vi "Autonomous Independent.vi"() -> ()   [LabVIEW 2015]
doc: "This VI is called when autonomous begins, and will automatically be terminated when autonomous ends. You can carry out timed or sensor driven robot movement independently without needing to return to the caller."
uses:
  <vilib>/Rock Robotics/WPI/Utilities/WPI_GetSetVariantRefNum.vi
  <vilib>/Rock Robotics/Network Tables/NT Read String.vi
  <vilib>/Rock Robotics/WPI/RobotDrive/WPI_RobotDriveArcadeDrive_Standard(NoSaturation).vi
  <vilib>/Rock Robotics/Network Tables/NT Write Numeric Array.vi
panel:
  out "Current Movement, for debugging":T1 {"Y Joystick Value" scale=1.0..-1.0; "X Joystick Value" scale=-1.0..1.0}
  in  "Array of robot movements":T2(array[cluster])=[{"X Joystick Value"=0.39393939393939403, "Y Joystick Value"=0.0, "Delay (sec)"=1.0, "Movement Name"="turn"}, {"X Joystick Value"=-0.3737373737373737, "Y Joystick Value"=0.0, "Delay (sec)"=1.0, "Movement Name"="turn back"}] {"Y Joystick Value" scale=1.0..-1.0; "X Joystick Value" scale=-1.0..1.0}
  # "Be sure to right-click and choose Data Operations>>Make Current Value default if you want to save the array values with the VI"
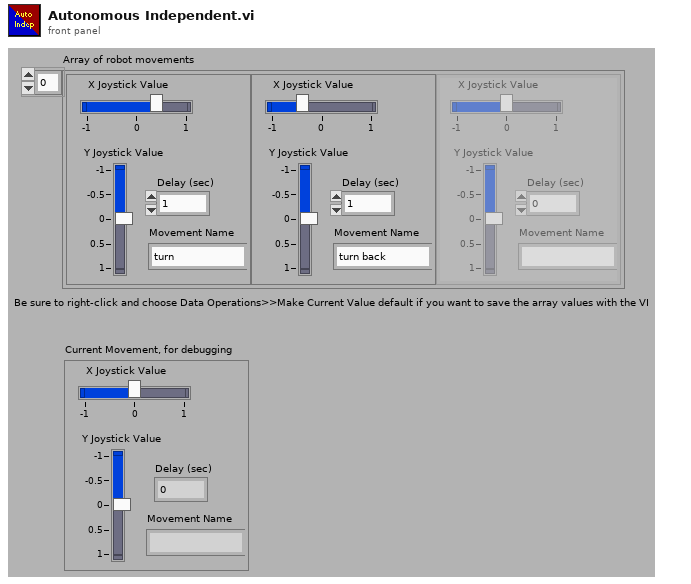
[diagram p1: front panel]
types:
  T1 = cluster{"X Joystick Value":dbl, "Y Joystick Value":dbl, "Delay (sec)":dbl, "Movement Name":string}
  T2 = cluster{"X Joystick Value":dbl, "Y Joystick Value":dbl, "Delay (sec)":dbl, "Movement Name":string}[]
  T3 = typedef "WPI_JoystickDevRef.ctl" = cluster{"Device":T4}
  T4 = typedef "WPI_JoystickDeviceEnum.ctl" = enum16{"USB 0", "USB 1", "USB 2", "USB 3", "USB 4", "USB 5"}
  T5 = typedef "WPI_RobotDriveDevRef.ctl" = cluster{"DevStatus":errorcluster, "Motors[]":T6[], "Square Inputs":bool, "Max Output":dbl}
  T6 = typedef "WPI_MotorControlDeviceRef.ctl" = cluster{"DeviceStatus":errorcluster, "Type":T7, "PWM":cluster{"PWM Channel":T8, "DeadBand":T9}, "CAN":cluster{"Device Number":u8, "Control Mode":T10, "Semaphore":T11, "Max Vout":dbl, "TalonSRX Control Mode":T12}, "Invert":bool}
  T7 = typedef "WPI_MotorControlType.ctl" = enum16{"PWM", "CAN", "CANTalonSRX"}
  T8 = typedef "FPGA_DIOPWMChannel.ctl" = enum8{"PWM 0", "PWM 1", "PWM 2", "PWM 3", "PWM 4", "PWM 5", "PWM 6", "PWM 7", "PWM 8", "PWM 9", "PWM MXP 0", "PWM MXP 1", "PWM MXP 2", "PWM MXP 3", "PWM MXP 4", "PWM MXP 5", "PWM MXP 6", "PWM MXP 7", "PWM MXP 8", "PWM MXP 9", "Invalid"}
  T9 = typedef "WPI_PWMDeadband.ctl" = cluster{"Name":string, "maxPositivePwm":i32, "minPositivePwm":i32, "centerPwm":i32, "maxNegativePwm":i32, "minNegativePwm":i32, "angularRange":u16}
  T10 = typedef "WPI_CANJaguar_ControlMode.ctl" = enum8{"Percent VBus", "Current", "Speed", "Position", "Voltage"}
  T11 = typedef "Semaphore RefNum" = refnum<k1>
  T12 = typedef "WPI_CANTalonSRX_APIControlMode.ctl" = enum8{"Percent VBus", "Speed", "Position", "Slave", "Unchanged / Invalid", "Voltage Compensation", "Current", "Motion Profile"}
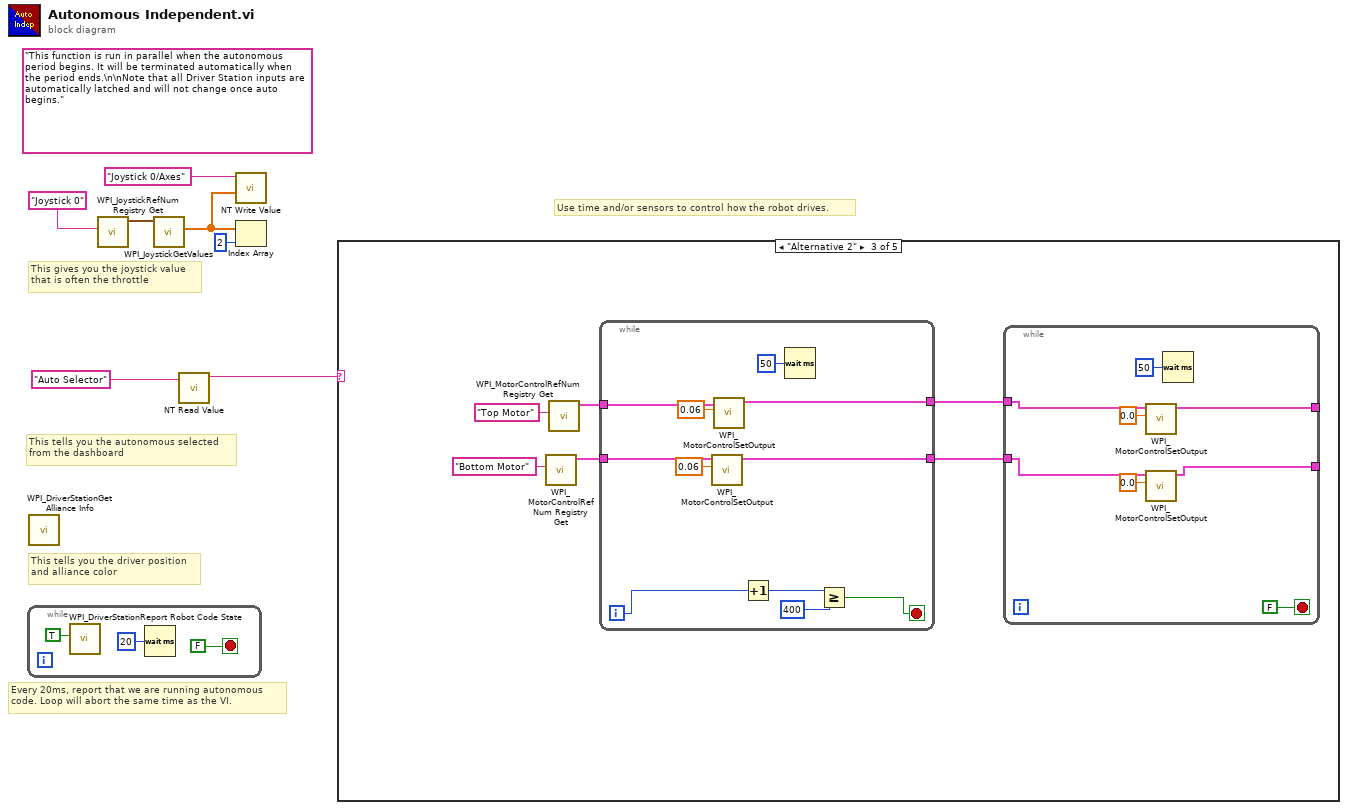
[diagram p0: block diagram]
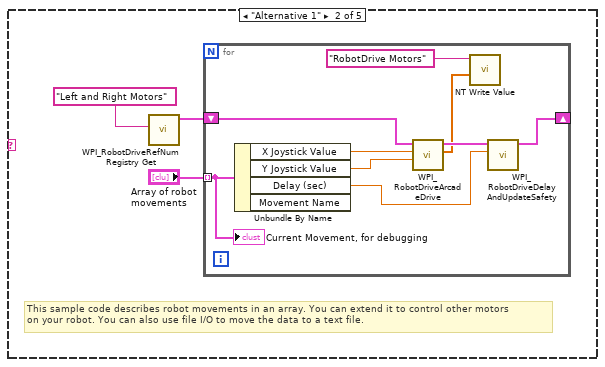
[diagram p3: hidden frame]
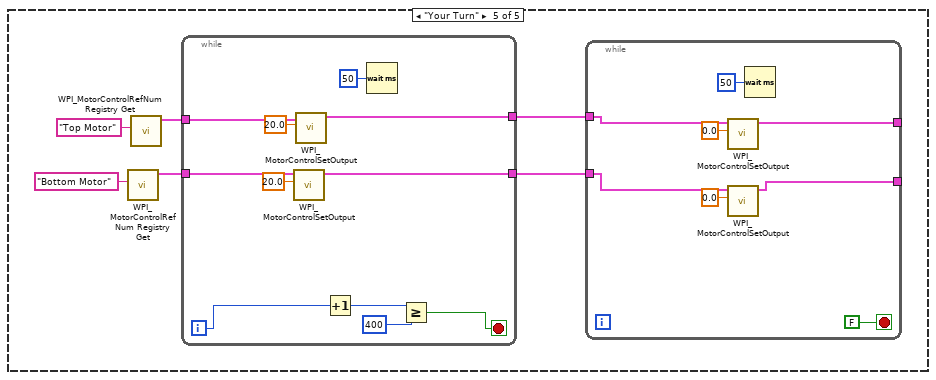
[diagram p5: hidden frame]
diagram:
  (unwired) "This function is run in parallel when the autonomous period begins. It will be terminated automatically when the period ends.\n\nNote that all Driver Station inputs are automatically latched and will not change once auto begins."
  # "This tells you the autonomous selected\nfrom the dashboard"
  # "Every 20ms, report that we are running autonomous\ncode. Loop will abort the same time as the VI."
  # "This gives you the joystick value\nthat is often the throttle"
  # "Use time and/or sensors to control how the robot drives."
  # "This tells you the driver position\nand alliance color"
  n1 = while {
    stop <- FALSE stop-if-true
    n2 = call <vilib>:"WPI_DriverStationReport Robot Code State.vi"("Autonomous"=TRUE) -> ()  [unwired: 10 in, 1 out]
    n3 = Wait (ms)(milliseconds to wait=u32 20) -> ()  [unwired: 1 out]
  }
  n4 = call <vilib>:"WPI_DriverStationGet Alliance Info.vi"() -> ()  [unwired: 12 out]
  n5 = call <vilib>:"WPI_JoystickRefNum Registry Get.vi"("refnum name"="Joystick 0") -> ("JoystickDevRef"=w6:T3)  [unwired: 1 in, 9 out]
  n6 = call <vilib>:"WPI_JoystickGetValues.vi"("JoystickDevRef"=w6) -> ("Axes"=w2:dbl[])  [unwired: 6 in, 4 out]
  n7 = call-poly <vilib>:"NT Read Value.vi"("Name"="Auto Selector") -> ("String"=w3:string)  [unwired: 9 in, 1 out]
  n8 = call-poly <vilib>:"NT Write Value.vi"("Numeric Array"=w2, "Name"="Joystick 0/Axes") -> ()  [unwired: 9 in, 1 out]
  n9 = Index Array(array=w2, index=2) -> ()  [unwired: 1 out]
  n10 = case shown="\"Alternative 2\"" w3 {
    frame Default {
      # "You can put your main auto here, or you can right-click on the case and make any\nother frame be the default case."
      # "This is the frame that will execute if no selection is made, or if it is not recognized"
    }
    frame "Alternative 1" {
      # "This sample code describes robot movements in an array. You can extend it to control other motors\non your robot. You can also use file I/O to move the data to a text file."
      n11 = call <vilib>:"WPI_RobotDriveRefNum Registry Get.vi"("refnum name"="Left and Right Motors") -> ("RobotDriveDevRef"=w12:T5)  [unwired: 1 in, 9 out]
      n12 = for {
        shift-right: [w20] -> _
        shift-left: w12 -> [w21]
        tunnel: "Array of robot movements" -> [w16] mode=indexing
        n13 = Unbundle By Name(w16) -> ("X Joystick Value"=w19:dbl, "Y Joystick Value"=w18:dbl, "Delay (sec)"=w17:dbl)  [unwired: 1 out]
        n14 = call-poly <vilib>:"WPI_RobotDriveArcadeDrive.vi"("Y axis value"=w18, "X axis value"=w19, "RobotDriveDevRef"=w21) -> ("Motor Values"=w14:dbl[], "RobotDriveDevRef"=w22:T5)  [unwired: 1 in, 6 out]
        n15 = call-poly <vilib>:"NT Write Value.vi"("Numeric Array"=w14, "Name"="RobotDrive Motors") -> ()  [unwired: 9 in, 1 out]
        n16 = call <vilib>:"WPI_RobotDriveDelayAndUpdateSafety.vi"("Delay (s)"=w17, "RobotDriveDevRef"=w22) -> ("RobotDriveDevRef 2"=w20:T5)  [unwired: 8 in, 1 out]
        "Current Movement, for debugging" <- w16
      }
    }
    frame "Alternative 2" {
      n17 = call <vilib>:"WPI_MotorControlRefNum Registry Get.vi"("refnum name"="Bottom Motor") -> ("MotorControlDevRef"=w28:T6)  [unwired: 9 in, 1 out]
      n18 = call <vilib>:"WPI_MotorControlRefNum Registry Get.vi"("refnum name"="Top Motor") -> ("MotorControlDevRef"=w27:T6)  [unwired: 9 in, 1 out]
      n19 = while {
        tunnel: w28 -> [w47]
        tunnel: w27 -> [w46]
        tunnel: [w40] -> w24
        tunnel: [w39] -> w23
        i -> [w42]
        stop <- w43 stop-if-true
        n20 = call <vilib>:"WPI_MotorControlSetOutput.vi"("Output"=0.06, "MotorControlDevRef"=w47) -> ("MotorControlDevRef"=w39:T6)  [unwired: 7 in, 2 out]
        n21 = call <vilib>:"WPI_MotorControlSetOutput.vi"("Output"=0.06, "MotorControlDevRef"=w46) -> ("MotorControlDevRef"=w40:T6)  [unwired: 7 in, 2 out]
        n22 = Increment(x=w42) -> (x+1=w44:i32)
        n23 = Wait (ms)(milliseconds to wait=u32 50) -> ()  [unwired: 1 out]
        n24 = Greater Or Equal?(x=w44, y=400) -> (x >= y?=w43:bool)
      }
      n25 = while {
        tunnel: w24 -> [w34]
        tunnel: w23 -> [w32]
        tunnel: [w33] -> _
        tunnel: [w31] -> _
        stop <- FALSE stop-if-true
        n26 = call <vilib>:"WPI_MotorControlSetOutput.vi"("Output"=0.0, "MotorControlDevRef"=w34) -> ("MotorControlDevRef"=w33:T6)  [unwired: 7 in, 2 out]
        n27 = call <vilib>:"WPI_MotorControlSetOutput.vi"("Output"=0.0, "MotorControlDevRef"=w32) -> ("MotorControlDevRef"=w31:T6)  [unwired: 7 in, 2 out]
        n28 = Wait (ms)(milliseconds to wait=u32 50) -> ()  [unwired: 1 out]
      }
    }
    frame "Alternative 3" {
    }
    frame "Your Turn" {
      n29 = call <vilib>:"WPI_MotorControlRefNum Registry Get.vi"("refnum name"="Bottom Motor") -> ("MotorControlDevRef"=w53:T6)  [unwired: 9 in, 1 out]
      n30 = call <vilib>:"WPI_MotorControlRefNum Registry Get.vi"("refnum name"="Top Motor") -> ("MotorControlDevRef"=w52:T6)  [unwired: 9 in, 1 out]
      n31 = while {
        tunnel: w53 -> [w72]
        tunnel: w52 -> [w71]
        tunnel: [w65] -> w49
        tunnel: [w64] -> w48
        i -> [w67]
        stop <- w68 stop-if-true
        n32 = call <vilib>:"WPI_MotorControlSetOutput.vi"("Output"=20.0, "MotorControlDevRef"=w72) -> ("MotorControlDevRef"=w64:T6)  [unwired: 7 in, 2 out]
        n33 = call <vilib>:"WPI_MotorControlSetOutput.vi"("Output"=20.0, "MotorControlDevRef"=w71) -> ("MotorControlDevRef"=w65:T6)  [unwired: 7 in, 2 out]
        n34 = Increment(x=w67) -> (x+1=w69:i32)
        n35 = Wait (ms)(milliseconds to wait=u32 50) -> ()  [unwired: 1 out]
        n36 = Greater Or Equal?(x=w69, y=400) -> (x >= y?=w68:bool)
      }
      n37 = while {
        tunnel: w49 -> [w59]
        tunnel: w48 -> [w57]
        tunnel: [w58] -> _
        tunnel: [w56] -> _
        stop <- FALSE stop-if-true
        n38 = call <vilib>:"WPI_MotorControlSetOutput.vi"("Output"=0.0, "MotorControlDevRef"=w59) -> ("MotorControlDevRef"=w58:T6)  [unwired: 7 in, 2 out]
        n39 = call <vilib>:"WPI_MotorControlSetOutput.vi"("Output"=0.0, "MotorControlDevRef"=w57) -> ("MotorControlDevRef"=w56:T6)  [unwired: 7 in, 2 out]
        n40 = Wait (ms)(milliseconds to wait=u32 50) -> ()  [unwired: 1 out]
      }
    }
  }
